vi "Read Agent Public Key Data.vi"(8 "error in (no error)":errorcluster, 11 "agent public key":T2) -> (0 "error out":errorcluster, 2 "value":T1)   [LabVIEW 2013, in "libssh2.lvlib"]
doc: "Returns data associated with <B>agent public key</B>."
uses:
  libssh2.lvlib
  Agent Public Key Refnum.ctl
  libssh2_agent_publickey.ctl
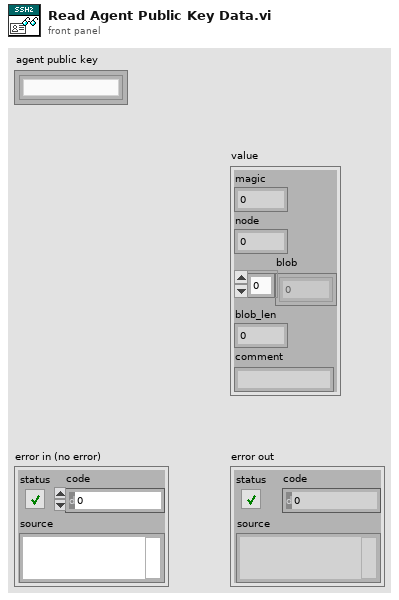
[diagram p1: front panel]
types:
  T1 = typedef "libssh2.lvlib/libssh2_agent_publickey.ctl" = cluster{"magic":i32, "node":u64, "blob":u8[], "blob_len":i32, "comment":string}
  T2 = typedef "libssh2.lvlib/Agent Public Key Refnum.ctl" = refnum<k1>
  T3 = cluster{"magic":u32, "node":u32, "blob":u32, "blob_len":u32, "comment":u32}
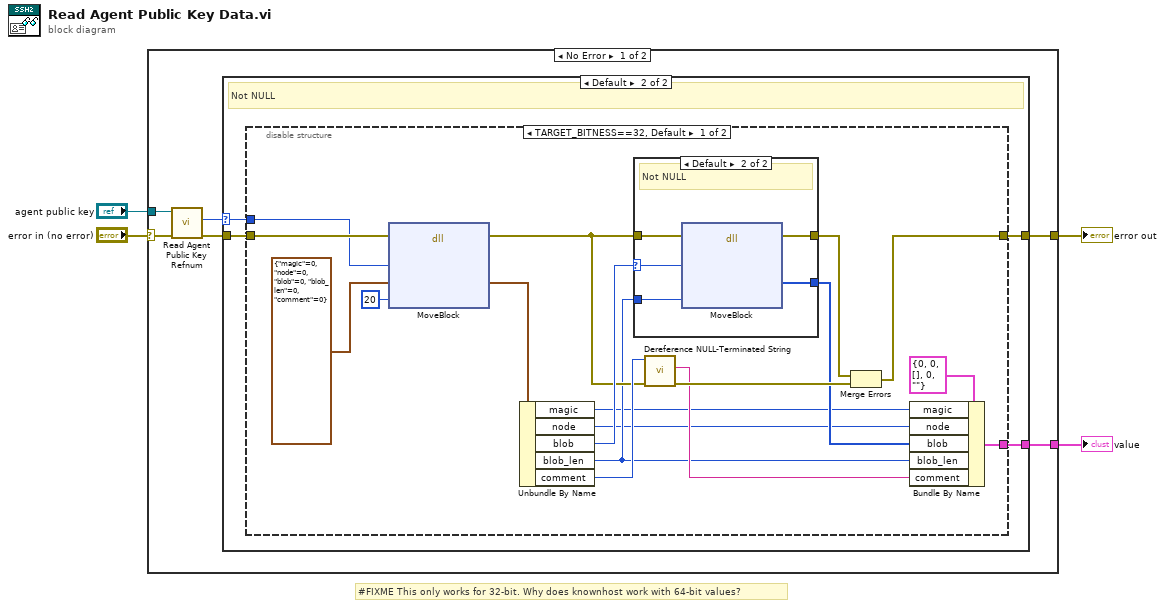
[diagram p0: block diagram]
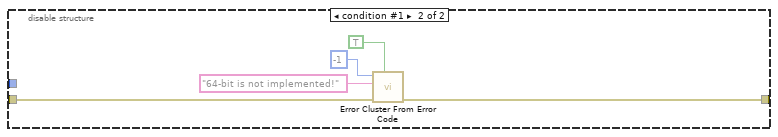
[diagram p4: hidden frame]
diagram:
  # "#FIXME This only works for 32-bit. Why does knownhost work with 64-bit values?"
  n1 = case shown="No Error" "error in (no error)" {
    selector: "error in (no error)" -> [w6 w44]
    tunnel: "agent public key" -> [w10 _]
    tunnel: [w8 w44] -> w3
    tunnel: [w5 _] -> w1
    frame No Error {
      n2 = call "Read Agent Public Key Refnum.vi"("error in (no error)"=w6, "agent public key"=w10) -> ("error out"=w9:errorcluster, "libssh2_agent_publickey*"=w7:u64)  [unwired: 8 in]
      n3 = case shown="Default" w7 {
        selector: w7 -> [_ w13]
        tunnel: w9 -> [w11 w15]
        tunnel: [w11 w14] -> w8
        tunnel: [_ w12] -> w5
        frame 0 {
          # "NULL"
        }
        frame Default {
          # "Not NULL"
          n4 = disable-structure shown="TARGET_BITNESS==32, Default" {
            disable-tunnel: w15 -> [w33 w43]
            disable-tunnel: [w29 w42] -> w14
            disable-tunnel: w13 -> [w28 _]
            disable-tunnel: [w20 _] -> w12
            frame condition #0 (active) {
              n5 = dll-call lib="LabVIEW" fn="MoveBlock"(error in=w33, "ps"=w28, "pd"=T3 {"magic"=0, "node"=0, "blob"=0, "blob_len"=0, "comment"=0}, "size"=i64 20) -> (error out=w25:errorcluster, "pd"=w23:T3)  [unwired: 5 in, 1 out]
              n6 = Unbundle By Name(w23) -> ("magic"=w16:u32, "node"=w17:u32, "blob"=w27:u32, "blob_len"=w18:u32, "comment"=w26:u32)
              n7 = case shown="Default" w27 {
                selector: w27 -> [_ w35]
                tunnel: w18 -> [_ w38]
                tunnel: [_ w37] -> w19
                tunnel: [_ w36] -> w30
                tunnel: w25 -> [_ w34]
                frame 0 {
                  # "NULL"
                }
                frame Default {
                  # "Not NULL"
                  n8 = dll-call lib="LabVIEW" fn="MoveBlock"(error in=w34, "ps"=w35, "size"=w38) -> (error out=w36:errorcluster, "pd"=w37:u8[])  [unwired: 6 in, 1 out]
                }
              }
              n9 = call "Dereference NULL-Terminated String.vi"("error in (no error)"=w25, "char*"=w26) -> ("error out"=w31:errorcluster, "string"=w21:string)  [unwired: 8 in]
              n10 = Merge Errors(w30, w31) -> (w29:errorcluster)
              n11 = Bundle By Name(cluster=T1 {"magic"=0, "node"=0, "blob"=[], "blob_len"=0, "comment"=""} ("libssh2_agent_publickey"), "magic"=w16, "node"=w17, "blob"=w19, "blob_len"=w18, "comment"=w21) -> (w20:T1)
            }
            frame condition #1 {
              n12 = call <vilib>:"Error Cluster From Error Code.vi"("show call chain? (False)"=TRUE, "error in (no error)"=w43, "error message (\"\")"="64-bit is not implemented!" ("error message (\"\")"), "error code (0)"=-1) -> ("error out"=w42:errorcluster)  [unwired: 5 in]
            }
          }
        }
      }
    }
    frame Error {
    }
  }
  "error out" <- w3
  "value" <- w1
